vi "calibracao_adq.vi"() -> ()   [LabVIEW 2019]
uses:
  <vilib>/Utility/file.llb/Read Delimited Spreadsheet (string).vi
  <vilib>/Utility/file.llb/Write Delimited Spreadsheet (string).vi
panel:
  in  "Valores reserva":T1
  in  "Valores":T1
  in  "Salvar":bool
  in  "Não alterar":bool
  in  "Padrão":bool
  in  "Iniciar \nCalibração":bool
  in  "stop":bool
  in  "STOP":bool
  # "MIN"
  # "MAX"
  # "P1"
  # "kPa"
  # "P2"
  # "kPa"
  # "P3"
  # "kPa"
  # "P4"
  # "kPa"
  # "Pfundo"
  # "kPa"
  # "MIN"
  # "MAX"
  # "P1"
  # "kPa"
  # "P2"
  # "kPa"
  # "P3"
  # "kPa"
  # "P4"
  # "kPa"
  # "Pfundo"
  # "kPa"
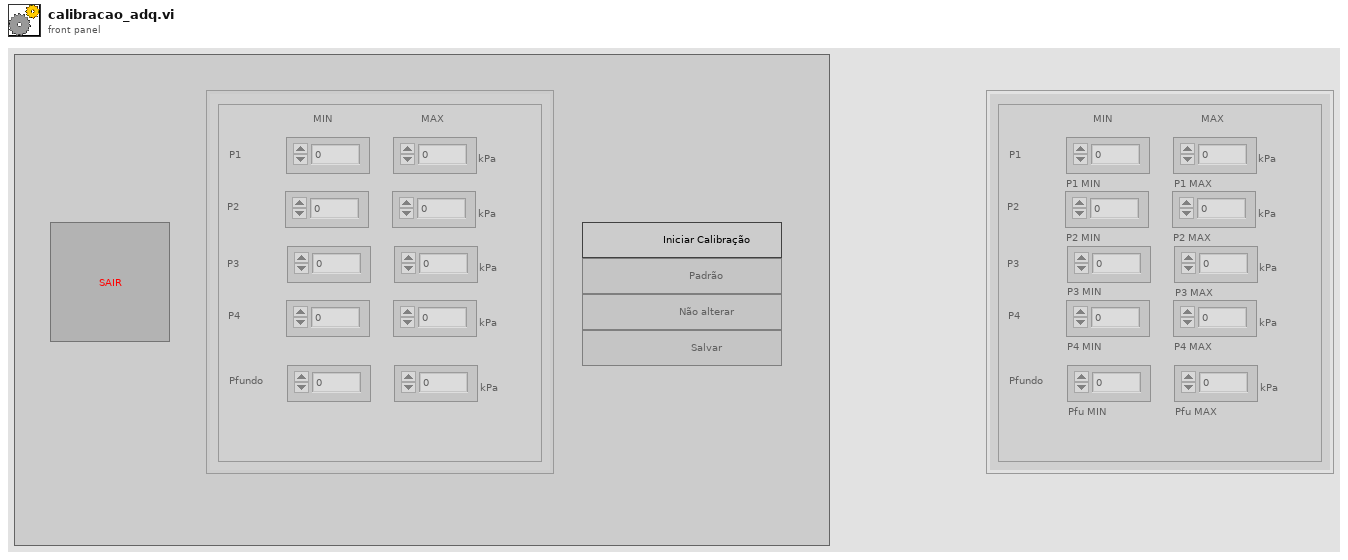
[diagram p1: front panel]
types:
  T1 = cluster{"P1 MIN":i32, "P1 MAX":i32, "P2 MIN":i32, "P2 MAX":i32, "P3 MIN":i32, "P3 MAX":i32, "P4 MIN":i32, "P4 MAX":i32, "Pfu MIN":i32, "Pfu MAX":i32}
  T2 = enum8{"Enabled", "Disabled", "Disabled and Grayed Out"}
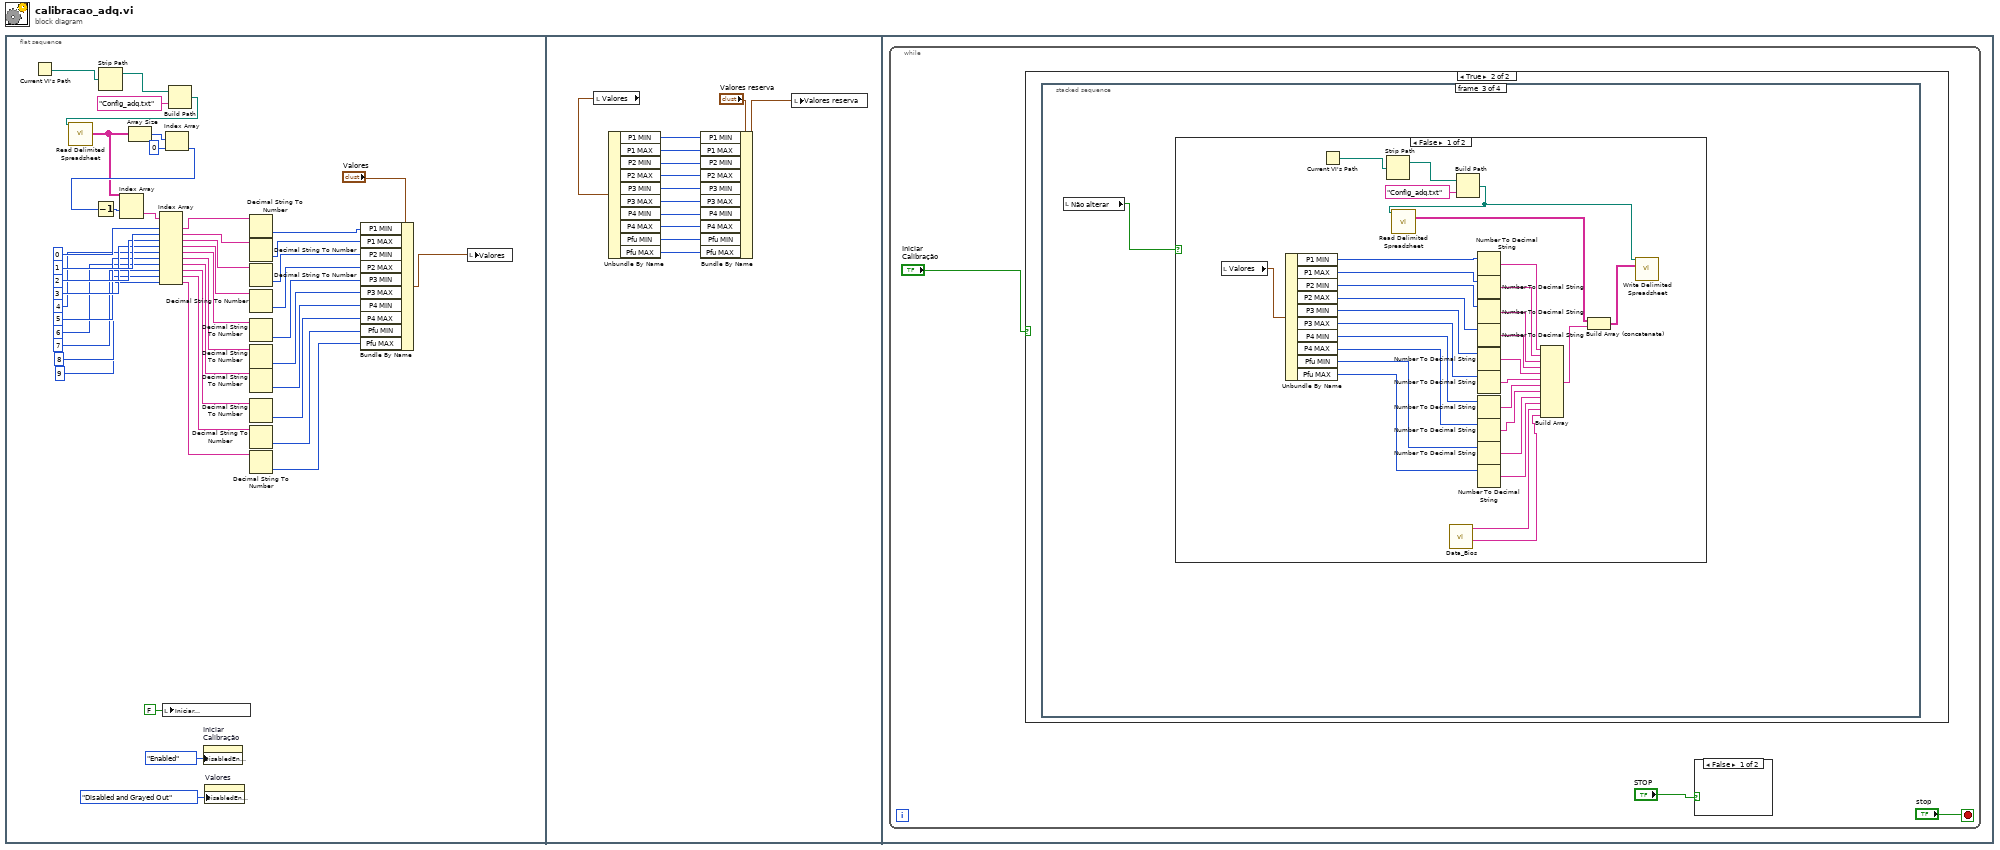
[diagram p0: block diagram]
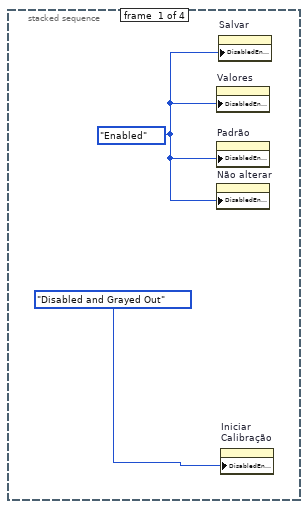
[diagram p3: hidden frame]
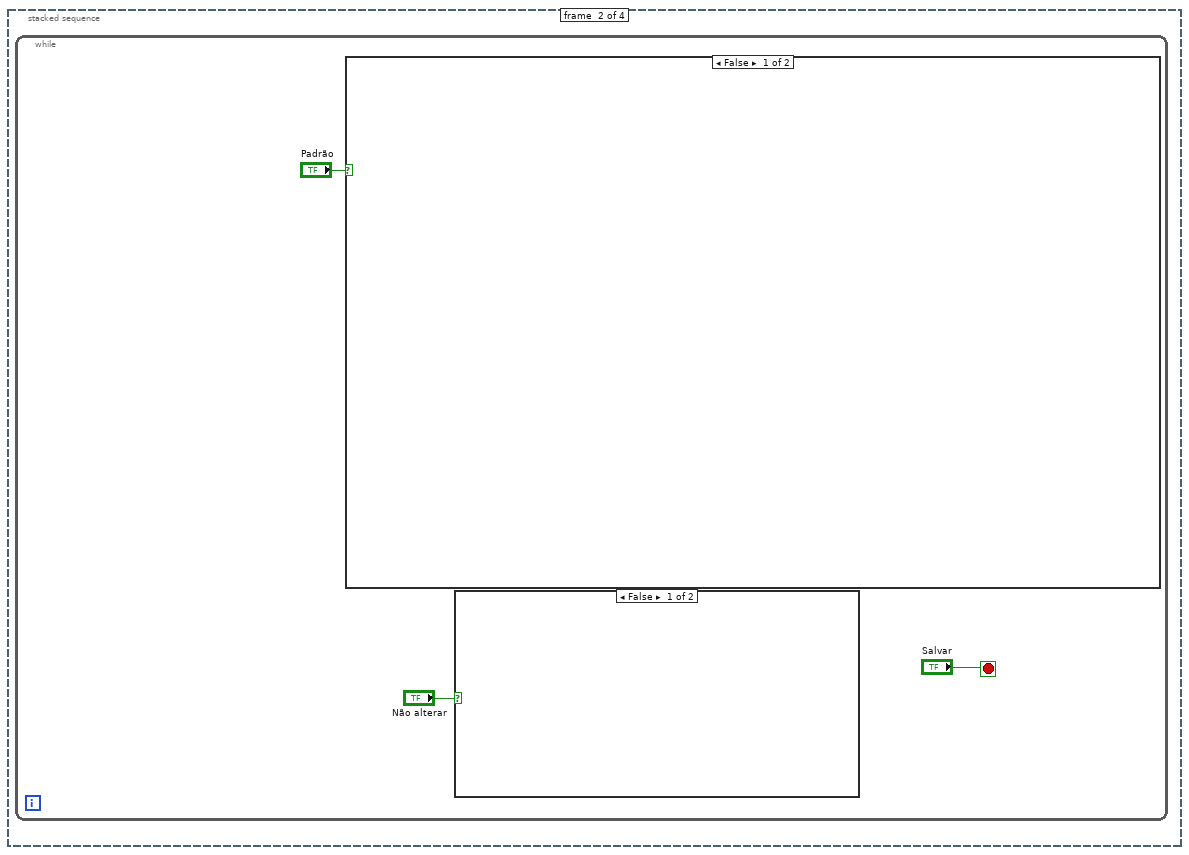
[diagram p4: hidden frame]
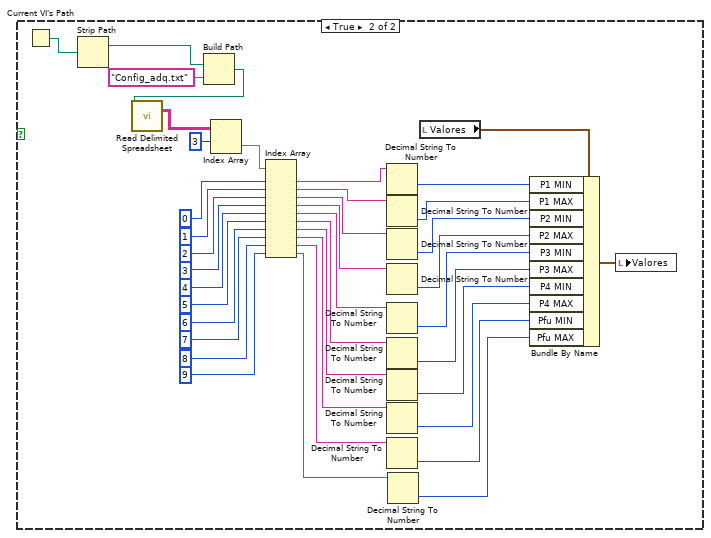
[diagram p5: hidden frame]
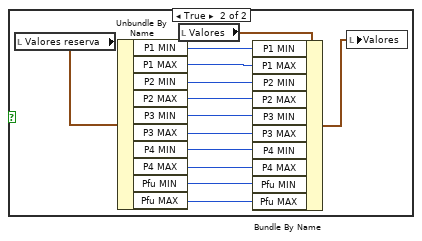
[diagram p6: hidden frame]
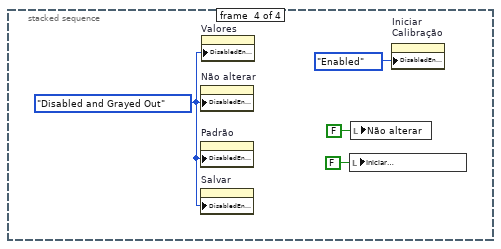
[diagram p8: hidden frame]
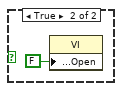
[diagram p9: hidden frame]
diagram:
  n1 = flat-sequence {
    frame #0 {
      n2 = Current VI's Path() -> (path=w27:path)
      n3 = Strip Path(path=w27) -> (stripped path=w26:path)  [unwired: 1 out]
      n4 = local write "Iniciar \nCalibração"(FALSE ("Iniciar \nCalibração")) -> ()
      n5 = Build Path(base path=w26, name or relative path="Config_adq.txt") -> (appended path=w24:path)
      n6 = call-poly <vilib>:"Read Delimited Spreadsheet.vi"("file path (dialog if empty)"=w24) -> ("all rows"=w30:string[][])  [unwired: 9 in, 5 out]
      n7 = Array Size(array=w30) -> (size(s)=w45:i32[])
      n8 = Index Array(array=w45, index=0) -> (element=w43:i32)
      n9 = Decrement(x=w43) -> (x-1=w42:i32)
      n10 = Index Array(array=w30, index (row)=w42) -> (element=w41:string[])  [unwired: 1 in]
      n11 = Index Array(array=w41, index #1=0 ("index"), index #2=1 ("index"), index #3=2 ("index"), index #4=3 ("index"), index #5=4 ("index"), index #6=5 ("index"), index #7=6 ("index"), index #8=7 ("index"), index #9=8 ("index"), index #10=9 ("index")) -> (element #1=w4:string, element #2=w36:string, element #3=w35:string, element #4=w34:string, element #5=w28:string, element #6=w23:string, element #7=w22:string, element #8=w21:string, element #9=w20:string, element #10=w2:string)
      n12 = property on="Iniciar \nCalibração" class="Bool (strict)"("DisabledEnum"=T2."Enabled" ("Disabled")) -> ()  [unwired: 2 in, 2 out]
      n13 = property on="Valores" class="Clust (strict)"("DisabledEnum"=T2."Disabled and Grayed Out" ("Disabled")) -> ()  [unwired: 2 in, 2 out]
      n14 = Decimal String To Number(string=w4) -> (number=w13:i32)  [unwired: 2 in, 1 out]
      n15 = Decimal String To Number(string=w36) -> (number=w12:i32)  [unwired: 2 in, 1 out]
      n16 = Decimal String To Number(string=w35) -> (number=w11:i32)  [unwired: 2 in, 1 out]
      n17 = Decimal String To Number(string=w34) -> (number=w10:i32)  [unwired: 2 in, 1 out]
      n18 = Decimal String To Number(string=w28) -> (number=w9:i32)  [unwired: 2 in, 1 out]
      n19 = Decimal String To Number(string=w23) -> (number=w8:i32)  [unwired: 2 in, 1 out]
      n20 = Decimal String To Number(string=w22) -> (number=w7:i32)  [unwired: 2 in, 1 out]
      n21 = Decimal String To Number(string=w21) -> (number=w6:i32)  [unwired: 2 in, 1 out]
      n22 = Decimal String To Number(string=w20) -> (number=w5:i32)  [unwired: 2 in, 1 out]
      n23 = Decimal String To Number(string=w2) -> (number=w1:i32)  [unwired: 2 in, 1 out]
      n24 = Bundle By Name(cluster="Valores", "P1 MIN"=w13, "P1 MAX"=w12, "P2 MIN"=w11, "P2 MAX"=w10, "P3 MIN"=w9, "P3 MAX"=w8, "P4 MIN"=w7, "P4 MAX"=w6, "Pfu MIN"=w5, "Pfu MAX"=w1) -> (w14:T1)
      n25 = local write "Valores"(w14) -> ()
    }
    frame #1 {
      n26 = local read "Valores"() -> (w58:T1)
      n27 = Unbundle By Name(w58) -> ("P1 MIN"=w55:i32, "P1 MAX"=w54:i32, "P2 MIN"=w53:i32, "P2 MAX"=w52:i32, "P3 MIN"=w51:i32, "P3 MAX"=w50:i32, "P4 MIN"=w49:i32, "P4 MAX"=w48:i32, "Pfu MIN"=w47:i32, "Pfu MAX"=w46:i32)
      n28 = Bundle By Name(cluster="Valores reserva", "P1 MIN"=w55, "P1 MAX"=w54, "P2 MIN"=w53, "P2 MAX"=w52, "P3 MIN"=w51, "P3 MAX"=w50, "P4 MIN"=w49, "P4 MAX"=w48, "Pfu MIN"=w47, "Pfu MAX"=w46) -> (w56:T1)
      n29 = local write "Valores reserva"(w56) -> ()
    }
    frame #2 {
      n30 = while {
        stop <- "stop" stop-if-true
        n31 = case shown="True" "Iniciar \nCalibração" {
          frame False {
          }
          frame True {
            n32 = stacked-sequence {
              frame #0 {
                w62 = T2."Enabled" ("Disabled")
                n33 = property on="Valores" class="Clust (strict)"("DisabledEnum"=w62) -> ()  [unwired: 2 in, 2 out]
                n34 = property on="Padrão" class="Bool"("DisabledEnum"=w62) -> ()  [unwired: 2 in, 2 out]
                n35 = property on="Não alterar" class="Bool (strict)"("DisabledEnum"=w62) -> ()  [unwired: 2 in, 2 out]
                n36 = property on="Salvar" class="Bool"("DisabledEnum"=w62) -> ()  [unwired: 2 in, 2 out]
                n37 = property on="Iniciar \nCalibração" class="Bool (strict)"("DisabledEnum"=T2."Disabled and Grayed Out" ("Disabled")) -> ()  [unwired: 2 in, 2 out]
              }
              frame #1 {
                n38 = while {
                  stop <- "Salvar" stop-if-true
                  n39 = case shown="False" "Padrão" {
                    frame False {
                    }
                    frame True {
                      n40 = Current VI's Path() -> (path=w101:path)
                      n41 = Strip Path(path=w101) -> (stripped path=w100:path)  [unwired: 1 out]
                      n42 = Build Path(base path=w100, name or relative path="Config_adq.txt") -> (appended path=w102:path)
                      n43 = call-poly <vilib>:"Read Delimited Spreadsheet.vi"("file path (dialog if empty)"=w102) -> ("all rows"=w105:string[][])  [unwired: 9 in, 5 out]
                      n44 = Index Array(array=w105, index (row)=3) -> (element=w82:string[])  [unwired: 1 in]
                      n45 = Index Array(array=w82, index #1=0 ("index"), index #2=1 ("index"), index #3=2 ("index"), index #4=3 ("index"), index #5=4 ("index"), index #6=5 ("index"), index #7=6 ("index"), index #8=7 ("index"), index #9=8 ("index"), index #10=9 ("index")) -> (element #1=w81:string, element #2=w95:string, element #3=w94:string, element #4=w93:string, element #5=w91:string, element #6=w90:string, element #7=w89:string, element #8=w88:string, element #9=w87:string, element #10=w69:string)
                      n46 = Decimal String To Number(string=w81) -> (number=w79:i32)  [unwired: 2 in, 1 out]
                      n47 = Decimal String To Number(string=w95) -> (number=w78:i32)  [unwired: 2 in, 1 out]
                      n48 = Decimal String To Number(string=w94) -> (number=w77:i32)  [unwired: 2 in, 1 out]
                      n49 = Decimal String To Number(string=w93) -> (number=w76:i32)  [unwired: 2 in, 1 out]
                      n50 = Decimal String To Number(string=w91) -> (number=w75:i32)  [unwired: 2 in, 1 out]
                      n51 = Decimal String To Number(string=w90) -> (number=w74:i32)  [unwired: 2 in, 1 out]
                      n52 = Decimal String To Number(string=w89) -> (number=w73:i32)  [unwired: 2 in, 1 out]
                      n53 = Decimal String To Number(string=w88) -> (number=w72:i32)  [unwired: 2 in, 1 out]
                      n54 = Decimal String To Number(string=w87) -> (number=w71:i32)  [unwired: 2 in, 1 out]
                      n55 = Decimal String To Number(string=w69) -> (number=w68:i32)  [unwired: 2 in, 1 out]
                      n56 = local read "Valores"() -> (w80:T1)
                      n57 = Bundle By Name(cluster=w80, "P1 MIN"=w79, "P1 MAX"=w78, "P2 MIN"=w77, "P2 MAX"=w76, "P3 MIN"=w75, "P3 MAX"=w74, "P4 MIN"=w73, "P4 MAX"=w72, "Pfu MIN"=w71, "Pfu MAX"=w68) -> (w67:T1)
                      n58 = local write "Valores"(w67) -> ()
                    }
                  }
                  n59 = case shown="False" "Não alterar" {
                    frame False {
                    }
                    frame True {
                      n60 = local read "Valores reserva"() -> (w118:T1)
                      n61 = Unbundle By Name(w118) -> ("P1 MIN"=w116:i32, "P1 MAX"=w115:i32, "P2 MIN"=w114:i32, "P2 MAX"=w113:i32, "P3 MIN"=w112:i32, "P3 MAX"=w111:i32, "P4 MIN"=w110:i32, "P4 MAX"=w109:i32, "Pfu MIN"=w108:i32, "Pfu MAX"=w107:i32)
                      n62 = local read "Valores"() -> (w117:T1)
                      n63 = Bundle By Name(cluster=w117, "P1 MIN"=w116, "P1 MAX"=w115, "P2 MIN"=w114, "P2 MAX"=w113, "P3 MIN"=w112, "P3 MAX"=w111, "P4 MIN"=w110, "P4 MAX"=w109, "Pfu MIN"=w108, "Pfu MAX"=w107) -> (w106:T1)
                      n64 = local write "Valores"(w106) -> ()
                    }
                  }
                }
              }
              frame #2 {
                n65 = local read "Não alterar"() -> (w119:bool)
                n66 = case shown="False" w119 {
                  frame False {
                    n67 = local read "Valores"() -> (w142:T1)
                    n68 = Unbundle By Name(w142) -> ("P1 MIN"=w141:i32, "P1 MAX"=w139:i32, "P2 MIN"=w138:i32, "P2 MAX"=w137:i32, "P3 MIN"=w136:i32, "P3 MAX"=w135:i32, "P4 MIN"=w134:i32, "P4 MAX"=w133:i32, "Pfu MIN"=w132:i32, "Pfu MAX"=w131:i32)
                    n69 = Current VI's Path() -> (path=w147:path)
                    n70 = Strip Path(path=w147) -> (stripped path=w146:path)  [unwired: 1 out]
                    n71 = call "Data_Bios.vi"() -> ("Hora"=w120:string, "Data"=w121:string)  [unwired: 8 in, 1 out]
                    n72 = Build Path(base path=w146, name or relative path="Config_adq.txt") -> (appended path=w144:path)
                    n73 = call-poly <vilib>:"Read Delimited Spreadsheet.vi"("file path (dialog if empty)"=w144) -> ("all rows"=w149:string[][])  [unwired: 9 in, 5 out]
                    n74 = Number To Decimal String(number=w141) -> (decimal integer string=w140:string)  [unwired: 1 in]
                    n75 = Number To Decimal String(number=w139) -> (decimal integer string=w130:string)  [unwired: 1 in]
                    n76 = Number To Decimal String(number=w138) -> (decimal integer string=w129:string)  [unwired: 1 in]
                    n77 = Number To Decimal String(number=w137) -> (decimal integer string=w128:string)  [unwired: 1 in]
                    n78 = Number To Decimal String(number=w136) -> (decimal integer string=w127:string)  [unwired: 1 in]
                    n79 = Number To Decimal String(number=w135) -> (decimal integer string=w126:string)  [unwired: 1 in]
                    n80 = Number To Decimal String(number=w134) -> (decimal integer string=w125:string)  [unwired: 1 in]
                    n81 = Number To Decimal String(number=w133) -> (decimal integer string=w124:string)  [unwired: 1 in]
                    n82 = Number To Decimal String(number=w132) -> (decimal integer string=w123:string)  [unwired: 1 in]
                    n83 = Number To Decimal String(number=w131) -> (decimal integer string=w122:string)  [unwired: 1 in]
                    n84 = Build Array(w140, w130, w129, w128, w127, w126, w125, w124, w123, w122, w121, w120) -> (w143:string[])
                    n85 = Build Array (concatenate)(w149, w143) -> (w148:string[][])
                    n86 = call-poly <vilib>:"Write Delimited Spreadsheet.vi"("file path (dialog if empty)"=w144, "2D data"=w148) -> ()  [unwired: 12 in, 2 out]
                  }
                  frame True {
                  }
                }
              }
              frame #3 {
                w150 = T2."Disabled and Grayed Out" ("Disabled")
                n87 = property on="Não alterar" class="Bool (strict)"("DisabledEnum"=w150) -> ()  [unwired: 2 in, 2 out]
                n88 = property on="Padrão" class="Bool"("DisabledEnum"=w150) -> ()  [unwired: 2 in, 2 out]
                n89 = property on="Salvar" class="Bool"("DisabledEnum"=w150) -> ()  [unwired: 2 in, 2 out]
                n90 = property on="Valores" class="Clust (strict)"("DisabledEnum"=w150) -> ()  [unwired: 2 in, 2 out]
                n91 = local write "Iniciar \nCalibração"(FALSE ("Iniciar \nCalibração")) -> ()
                n92 = local write "Não alterar"(FALSE ("Não alterar")) -> ()
                n93 = property on="Iniciar \nCalibração" class="Bool (strict)"("DisabledEnum"=T2."Enabled" ("Disabled")) -> ()  [unwired: 2 in, 2 out]
              }
            }
          }
        }
        n94 = case shown="False" "STOP" {
          frame False {
          }
          frame True {
            n95 = property class="VI"("Front Panel.Open"=FALSE ("Front Panel Window:Open")) -> ()  [unwired: 2 in, 2 out]
          }
        }
      }
    }
  }
